vi "Dimension.vi"(8 "error in (no error)":errorcluster) -> (0 "error out":errorcluster, 2 "Width":i32, 3 "Height":i32)   [LabVIEW 2010]
uses:
  D:/BenjaminR Data/LabVIEW Code/Resize Windows/Screen Resolution/Dimension/ScreenRes.dll
  ScreenRes.dll
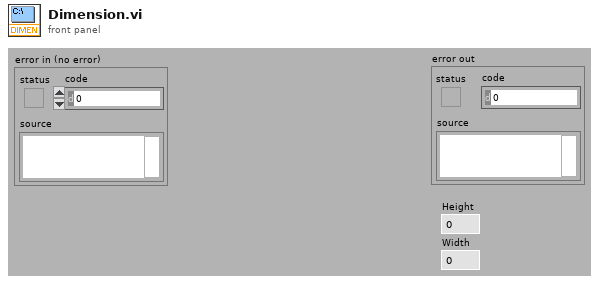
[diagram p1: front panel]
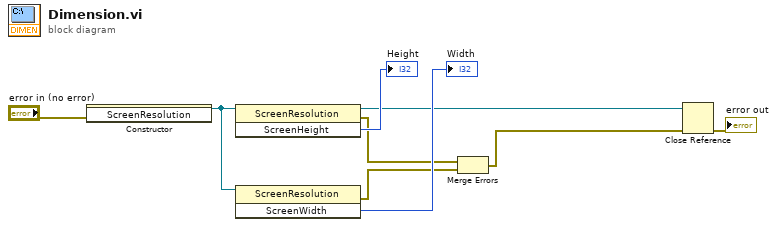
[diagram p0: block diagram]
diagram:
  n1 = constructor class="ScreenResolution"(error in="error in (no error)") -> (reference out=w9:refnum<k24>)  [unwired: 2 in, 2 out]
  n2 = invoke class="ScreenResolution" method="ScreenHeight"(reference=w9) -> (reference out=w2:refnum<k24>, error out=w3:errorcluster, "ScreenHeight"=→"Height":i32)  [unwired: 2 in]
  n3 = invoke class="ScreenResolution" method="ScreenWidth"(reference=w9) -> (error out=w5:errorcluster, "ScreenWidth"=→"Width":i32)  [unwired: 2 in, 1 out]
  n4 = Merge Errors(w3, w5) -> (w4:errorcluster)
  n5 = Close Reference(reference=w2, error in (no error)=w4) -> (error out=→"error out":errorcluster)
